vi "Graph.vi"(8 "error in (no error)":errorcluster, 10 "signal out":waveform(dbl), 11 "Generador in":refnum<class "Generador.lvclass">) -> (0 "error out":errorcluster, 3 "Generador out":refnum<class "Generador.lvclass">)   [LabVIEW 2020, in "Generador señal.lvlib" / "Generador.lvclass"]
uses:
  Generador.lvclass
  Generador.lvclass/Generador.ctl
  Text File/Text File Messages/Save Text Msg/Save Text Msg.lvclass/Save Text Msg.ctl
  <vilib>/ActorFramework/Message Enqueuer/Message Enqueuer.lvclass/Message Enqueuer.ctl
  <vilib>/ActorFramework/Message Enqueuer/Enqueue.vi
  Text File/Text File Messages/Save Text Msg/Save Text Msg.lvclass
  C:/Program Files (x86)/National Instruments/LabVIEW 2020/vi.lib/ActorFramework/Message/Message.lvclass
  <vilib>/ActorFramework/Message Priority Queue/Priority Enqueue.vi
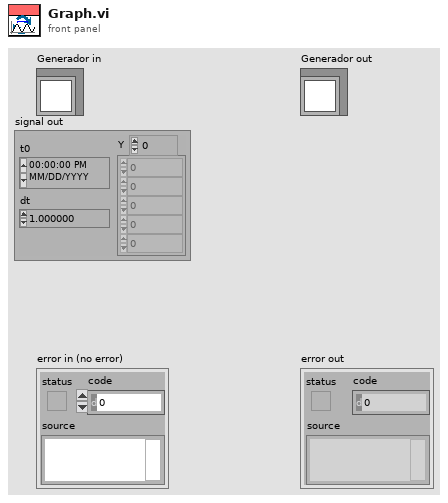
[diagram p1: front panel]
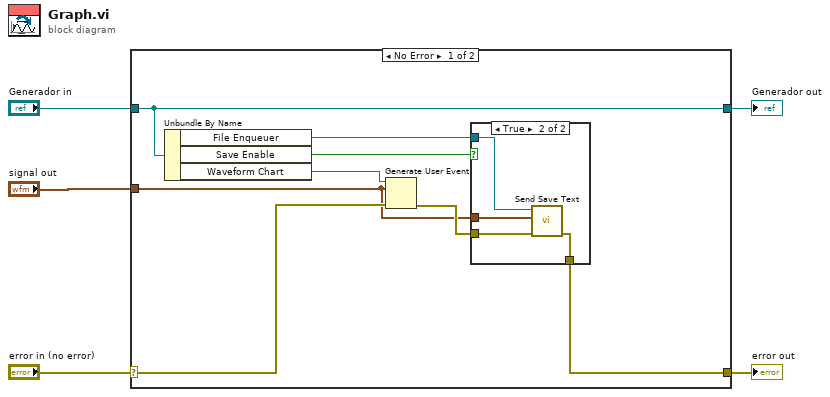
[diagram p0: block diagram]
diagram:
  n1 = case shown="No Error" "error in (no error)" {
    selector: "error in (no error)" -> [w11 w20]
    tunnel: [w9 w20] -> w4
    tunnel: [w13 w19] -> w2
    tunnel: "Generador in" -> [w13 w19]
    tunnel: "signal out" -> [w6 _]
    frame No Error {
      n2 = Unbundle By Name(w13) -> ("File Enqueuer"=w10:refnum<class "Message Enqueuer.lvclass">, "Save Enable"=w7:bool, "Waveform Chart"=w12:refnum<user-event>)
      n3 = Generate User Event(user event=w12, event data cluster=w6, error in=w11) -> (error out=w8:errorcluster)  [unwired: 1 in, 1 out]
      n4 = case shown="True" w7 {
        tunnel: w10 -> [_ w18]
        tunnel: [w14 w17] -> w9
        tunnel: w8 -> [w14 w16]
        tunnel: w6 -> [_ w15]
        frame False {
        }
        frame True {
          n5 = call "Send Save Text.vi"("error in (no error)"=w16, "Data"=w15, "Message Enqueuer"=w18) -> ("error out"=w17:errorcluster)  [unwired: 7 in, 1 out]
        }
      }
    }
    frame Error {
    }
  }
  "error out" <- w4
  "Generador out" <- w2
